vi "ArrayToExcel.vi"() -> ()   [LabVIEW 2020]
uses:
  <vilib>/Analysis/NI_AALBase.lvlib
panel:
  out "Grados":string[][](array[string])
  out "Guardar arreglos en Excel":dbl[][](graph)
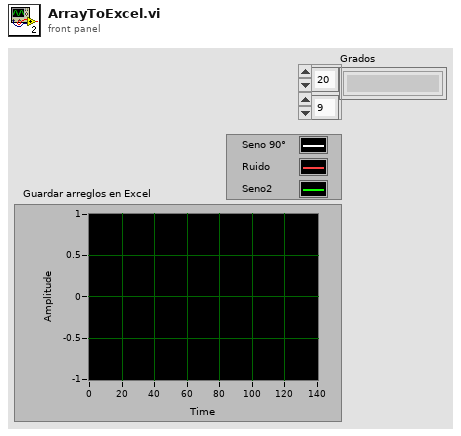
[diagram p1: front panel]
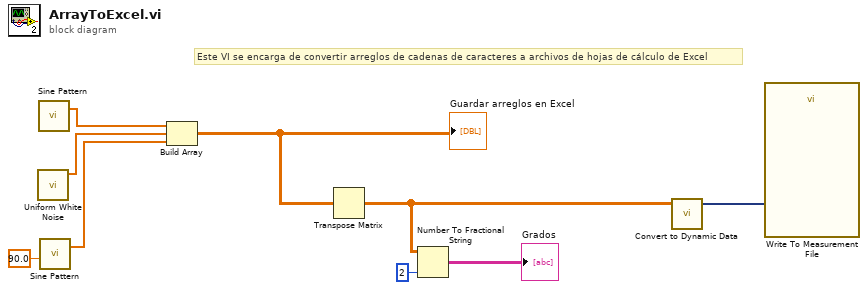
[diagram p0: block diagram]
diagram:
  # "Este VI se encarga de convertir arreglos de cadenas de caracteres a archivos de hojas de cálculo de Excel"
  n1 = call <vilib>:"Uniform White Noise.vi"() -> ("uniform white noise"=w6:dbl[])  [unwired: 10 in, 1 out]
  n2 = call <vilib>:"Sine Pattern.vi"() -> ("Sinusoidal Pattern"=w7:dbl[])  [unwired: 4 in, 1 out]
  n3 = call <vilib>:"Sine Pattern.vi"("phase(degrees)"=90.0) -> ("Sinusoidal Pattern"=w5:dbl[])  [unwired: 3 in, 1 out]
  n4 = Build Array(w7, w6, w5) -> (w4:dbl[][])
  "Guardar arreglos en Excel" <- w4
  n5 = Transpose Matrix(1:w4) -> (0:w2:dbl[][])
  n6 = Number To Fractional String(number=w2, precision (6)=i16 2) -> (F-format string=→"Grados":string[][])  [unwired: 2 in]
  n7 = call "Convert to Dynamic Data"("2D Array"=w2) -> ("Dynamic Data Type"=w1:dynamicdata)  [unwired: 3 in]
  n8 = call "Write To Measurement File"("Signals"=w1) -> ()  [unwired: 16 in, 3 out]
